vi "Filter.vi"(7 "sampling freq: fs":dbl=50000.0, 8 "error in (no error)":errorcluster, 9 "order":i32=2, 10 "low cutoff freq: fl":dbl=0.12500000000000006 format="%0.4f", 11 "Data_in":dynamicdata(graph)) -> (0 "error out":errorcluster, 3 "Data_out":dynamicdata(graph))   [LabVIEW 2012]
uses:
  <vilib>/Analysis/3filter.llb/Filter Passband Type.ctl
  <vilib>/Analysis/3filter.llb/Butterworth Filter (DBL).vi
  <vilib>/Analysis/NI_AALBase.lvlib
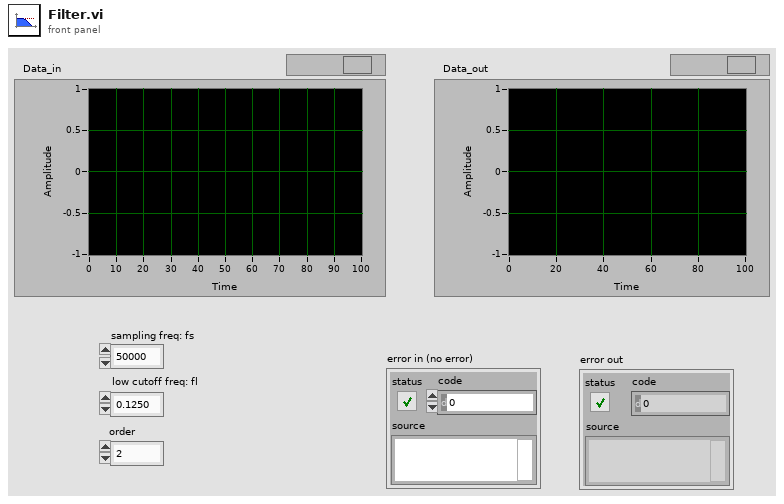
[diagram p1: front panel]
types:
  T1 = typedef "NI_AALBase.lvlib/Filter Passband Type.ctl" = enum32{"Lowpass", "Highpass", "Bandpass", "Bandstop"}
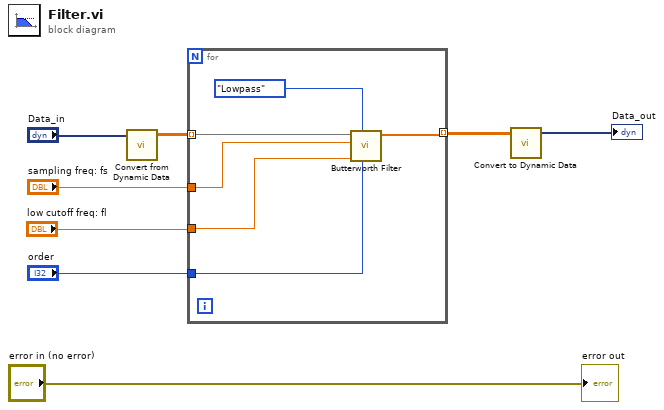
[diagram p0: block diagram]
diagram:
  n1 = call "Convert from Dynamic Data"("Dynamic Data Type"="Data_in") -> ("Array"=w8:dbl[][])  [unwired: 3 in]
  n2 = for {
    tunnel: [w14] -> w7 mode=indexing
    tunnel: "low cutoff freq: fl" -> [w13]
    tunnel: w8 -> [w11] mode=indexing
    tunnel: "order" -> [w10]
    tunnel: "sampling freq: fs" -> [w9]
    n3 = call-poly <vilib>:"Butterworth Filter.vi"("order"=w10, "filter type"=Filter_Passband_Type."Lowpass", "low cutoff freq: fl"=w13, "sampling freq: fs"=w9, "X"=w11) -> ("Filtered X"=w14:dbl[])  [unwired: 3 in, 1 out]
  }
  n4 = call "Convert to Dynamic Data"("2D Array"=w7) -> ("Dynamic Data Type"=→"Data_out":dynamicdata)  [unwired: 3 in]
  "error out" <- "error in (no error)"
